vi "task_msgQueue.vi"(8 "error in (no error)":errorcluster, 10 "ITaskChannel":refnum<class "ITaskChannel.lvclass">, 11 "ITask in":refnum<class "ITask.lvclass">) -> (0 "error out":errorcluster, 3 "ITask out":refnum<class "ITask.lvclass">)   [LabVIEW 2023]
uses:
  TLC_Daemon.lvlib
  ITask/ITask.lvclass
  ITaskChannel/ITaskChannel.lvclass
types:
  T1 = typedef "TLC_Daemon.lvlib/msg.ctl" = cluster{"message":string, "data":variant}
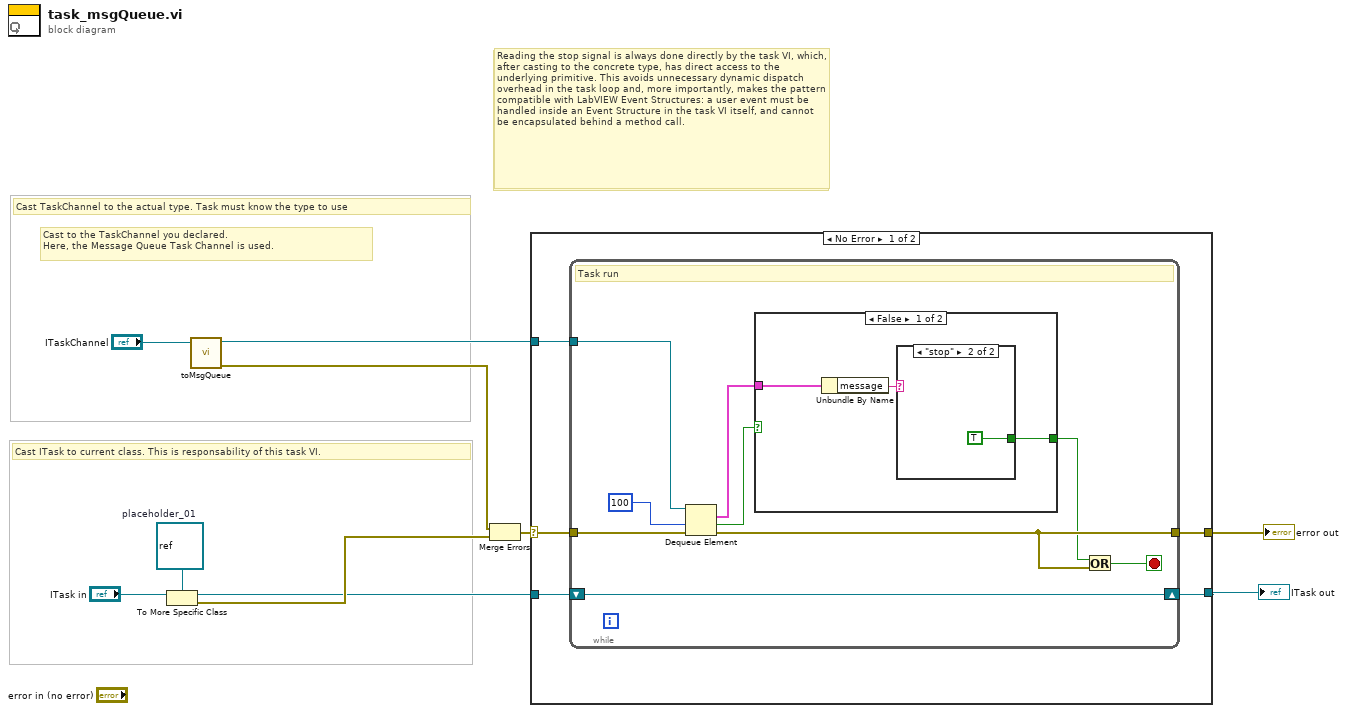
[diagram p0: block diagram]
diagram:
  w4 = refnum<class> refnum  # placeholder_01
  # "Cast to the TaskChannel you declared.\nHere, the Message Queue Task Channel is used."
  # "The stop signal is always handled directly by the task VI, which, after casting to the concrete type, has direct access to the underlying primitive. This avoids unnecessary dynamic dispatch overhead in the task loop and, more importantly, makes the pattern compatible with LabVIEW Event Structures: a user event must be handled inside an Event Structure in the task VI itself, and cannot be encapsulated behind a method call."
  # "Reading the stop signal is always done directly by the task VI, which, after casting to the concrete type, has direct access to the underlying primitive. This avoids unnecessary dynamic dispatch overhead in the task loop and, more importantly, makes the pattern compatible with LabVIEW Event Structures: a user event must be handled inside an Event Structure in the task VI itself, and cannot be encapsulated behind a method call."
  # "Cast ITask to current class. This is responsability of this task VI."
  # "Cast TaskChannel to the actual type. Task must know the type to use"
  n1 = To More Specific Class(target class=w4, reference="ITask in") -> (specific class reference=w8:refnum<class>, error out=w9:errorcluster)  [unwired: 1 in]
  n2 = call "toMsgQueue.vi"("ITaskChannel"="ITaskChannel") -> ("error out"=w1:errorcluster, "queueRef"=w2:refnum<queue>)  [unwired: 9 in]
  n3 = Merge Errors(w1, w9) -> (w6:errorcluster)
  n4 = case shown="No Error" w6 {
    selector: w6 -> [w14 w30]
    tunnel: w2 -> [w15 _]
    tunnel: w8 -> [w11 w29]
    tunnel: [w12 w29] -> w7
    tunnel: [w13 w30] -> w5
    frame No Error {
      n5 = while {
        tunnel: w15 -> [w24]
        tunnel: w14 -> [w22]
        tunnel: [w18] -> w13
        shift-right: [w21] -> w12
        shift-left: w11 -> [w21]
        stop <- w17 stop-if-true
        # "Task run"
        n6 = Dequeue Element(queue=w24, timeout in ms (-1)=100, error in (no error)=w22) -> (element=w19:T1, timed out?=w20:bool, error out=w18:errorcluster)  [unwired: 1 out]
        n7 = case shown="False" w20 {
          tunnel: w19 -> [w27 _]
          tunnel: [w25 _] -> w16
          frame False {
            n8 = Unbundle By Name(w27) -> ("message"=w26:string)
            n9 = case shown="\"stop\"" w26 {
              tunnel: [_ TRUE] -> w25
              frame "False", Default {
              }
              frame "stop" {
              }
            }
          }
          frame True {
          }
        }
        n10 = Or(x=w16, y=w18) -> (x .or. y?=w17:bool)
      }
    }
    frame Error {
    }
  }
  "error out" <- w5
  "ITask out" <- w7
